vi "stage and voice coil synchronization.vi"() -> ()   [LabVIEW 2020]
uses:
  <vilib>/DAQmx/create/channels.llb/DAQmx Create Channel (CO-Pulse Generation-Frequency).vi
  <vilib>/DAQmx/configure/timing.llb/DAQmx Timing (Implicit).vi
  <vilib>/DAQmx/create/channels.llb/DAQmx Create Channel (AO-Voltage-Basic).vi
  <vilib>/measure/NI_MABase.lvlib
  <vilib>/DAQmx/write.llb/DAQmx Write (Analog 2D DBL NChan NSamp).vi
  <vilib>/DAQmx/configure/timing.llb/DAQmx Timing (Use Waveform).vi
panel:
  out "size(s) 2":i32
  out "size(s)":i32
  out "last value outside of loop":dbl
  out "number of samples written per channel":u32
  in  "stop":bool
  out "Waveform Graph":waveform(dbl)[](graph)
  out "Number of slices":dbl
  in  "End position (mm)":dbl
  out "last value inside of loop":dbl
  out "Total Z thickness (mm)":dbl
  in  "Z slice width (mm)":dbl
  in  "Start position(mm)":dbl
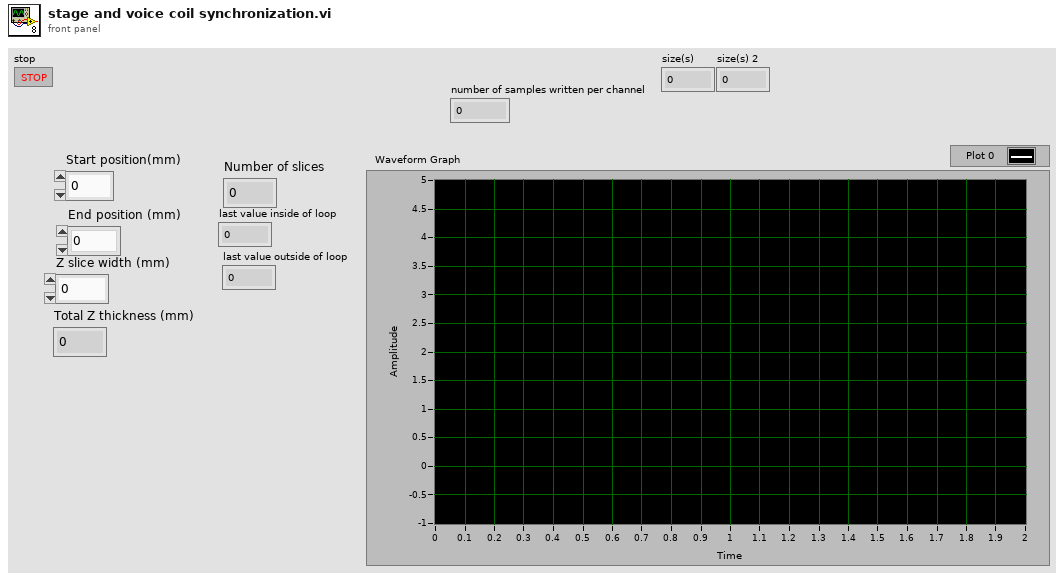
[diagram p1: front panel]
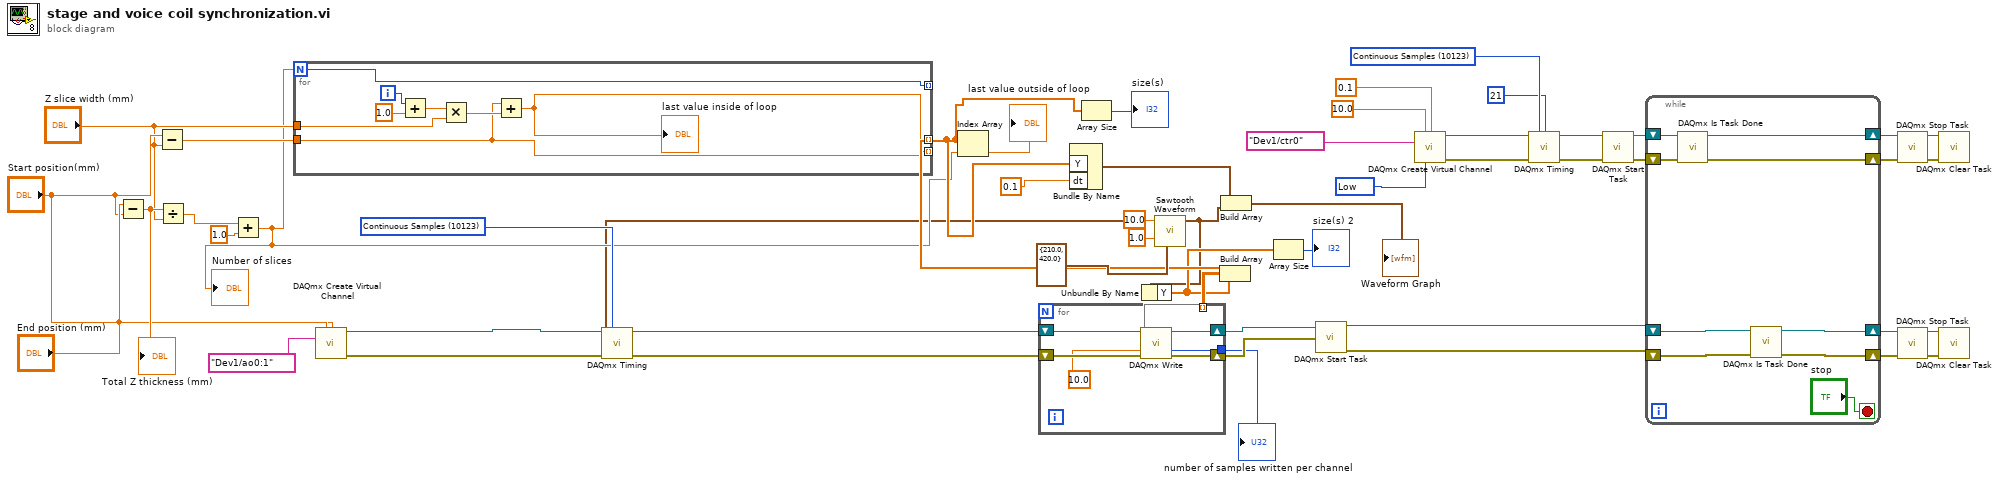
[diagram p0: block diagram]
diagram:
  w32 = 10214 items=["High"=10192, "Low"=10214] ("idle state")
  w34 = 10123 items=["Finite Samples"=10178, "Continuous Samples"=10123, "Hardware Timed Single Point"=12522] ("sample mode")
  w40 = 10123 items=["Finite Samples"=10178, "Continuous Samples"=10123, "Hardware Timed Single Point"=12522] ("sample mode")
  n1 = Subtract(x="End position (mm)", y="Start position(mm)") -> (x-y=w52:dbl)
  "Total Z thickness (mm)" <- w52
  n2 = Subtract(x="Start position(mm)", y="Z slice width (mm)") -> (x-y=w26:dbl)
  n3 = Divide(x=w52, y="Z slice width (mm)") -> (x/y=w5:dbl)
  n4 = Add(x=w5, y=1.0) -> (x+y=w2:dbl)
  "Number of slices" <- w2
  n5 = for {
    N: w2 -> [w55]
    tunnel: [w53] -> _ mode=indexing
    tunnel: "Z slice width (mm)" -> [w60]
    tunnel: [w54] -> w7 mode=indexing
    tunnel: [w55] -> _ mode=indexing
    tunnel: w26 -> [w53]
    i -> [w57]
    n6 = Add(x=w57, y=1.0) -> (x+y=w56:dbl)
    n7 = Multiply(x=w56, y=w60) -> (x*y=w59:dbl)
    n8 = Add(x=w53, y=w59) -> (x+y=w54:dbl)
    "last value inside of loop" <- w54
  }
  n9 = call-poly <vilib>:"DAQmx Create Virtual Channel.vi"("maximum value"="End position (mm)", "minimum value"="Start position(mm)", "physical channels"=tag "Dev1/ao0:1") -> ("task out"=w42:refnum<k21>, "error out"=w41:errorcluster)  [unwired: 11 in]
  n10 = Index Array "Index Array"(array=w7, index=w2) -> (element=→"last value outside of loop":dbl)
  n11 = Bundle By Name("Y"=w7, "dt"=0.1) -> (w14:waveform(dbl))  [unwired: 1 in]
  n12 = Array Size(array=w7) -> (size(s)=→"size(s)":i32)
  n13 = call <vilib>:"Sawtooth Waveform.vi"("sampling info"=cluster{"Fs":dbl, "#s":dbl} {"Fs"=210.0, "#s"=420.0}, "amplitude"=1.0, "frequency"=10.0) -> ("signal out"=w1:waveform(dbl))  [unwired: 7 in, 1 out]
  n14 = call-poly <vilib>:"DAQmx Timing.vi"("task/channels in"=w42, "sample mode"=w40, "waveform"=w1, "error in"=w41) -> ("task out"=w27:refnum<k21>, "error out"=w28:errorcluster)  [unwired: 10 in]
  n15 = Unbundle By Name(w1) -> ("Y"=w4:dbl[])
  n16 = Build Array(w7, w4) -> (w9:dbl[][])
  n17 = for {
    tunnel: [w62] -> w15
    tunnel: w9 -> [w61] mode=indexing
    shift-right: [w63] -> w16
    shift-left: w28 -> [w67]
    shift-right: [w64] -> w19
    shift-left: w27 -> [w66]
    n18 = call-poly <vilib>:"DAQmx Write.vi"("task/channels in"=w66, "data"=w61, "timeout"=10.0, "error in"=w67) -> ("task out"=w64:refnum<k21>, "number of samples written per channel"=w62:u32, "error out"=w63:errorcluster)  [unwired: 9 in]
  }
  "number of samples written per channel" <- w15
  n19 = Build Array(w14, w1) -> (→"Waveform Graph":waveform(dbl)[])
  n20 = Array Size(array=w4) -> (size(s)=→"size(s) 2":i32)
  n21 = call <vilib>:"DAQmx Start Task.vi"("task/channels in"=w19, "error in"=w16) -> ("task out"=w18:refnum<k21>, "error out"=w17:errorcluster)  [unwired: 12 in]
  n22 = call-poly <vilib>:"DAQmx Create Virtual Channel.vi"("frequency"=10.0, "duty cycle"=0.1, "counter"=tag "Dev1/ctr0", "idle state"=w32) -> ("task out"=w37:refnum<k21>, "error out"=w36:errorcluster)  [unwired: 10 in]
  n23 = call-poly <vilib>:"DAQmx Timing.vi"("task/channels in"=w37, "sample mode"=w34, "samples per channel"=21, "error in"=w36) -> ("task out"=w30:refnum<k21>, "error out"=w29:errorcluster)  [unwired: 10 in]
  n24 = call <vilib>:"DAQmx Start Task.vi"("task/channels in"=w30, "error in"=w29) -> ("task out"=w39:refnum<k21>, "error out"=w38:errorcluster)  [unwired: 12 in]
  n25 = while {
    shift-right: [w71] -> w44
    shift-left: w18 -> [w70]
    shift-right: [w74] -> w50
    shift-left: w39 -> [w76]
    shift-right: [w73] -> w48
    shift-left: w38 -> [w75]
    shift-right: [w72] -> w46
    shift-left: w17 -> [w69]
    stop <- "stop" stop-if-true
    n26 = call <vilib>:"DAQmx Is Task Done.vi"("task/channels in"=w76, "error in"=w75) -> ("task out"=w74:refnum<k21>, "error out"=w73:errorcluster)  [unwired: 11 in, 1 out]
    n27 = call <vilib>:"DAQmx Is Task Done.vi"("task/channels in"=w70, "error in"=w69) -> ("task out"=w71:refnum<k21>, "error out"=w72:errorcluster)  [unwired: 11 in, 1 out]
  }
  n28 = call <vilib>:"DAQmx Stop Task.vi"("task/channels in"=w50, "error in"=w48) -> ("task out"=w49:refnum<k21>, "error out"=w47:errorcluster)  [unwired: 12 in]
  n29 = call <vilib>:"DAQmx Stop Task.vi"("task/channels in"=w44, "error in"=w46) -> ("task out"=w43:refnum<k21>, "error out"=w45:errorcluster)  [unwired: 12 in]
  n30 = call <vilib>:"DAQmx Clear Task.vi"("task in"=w49, "error in"=w47) -> ()  [unwired: 13 in, 1 out]
  n31 = call <vilib>:"DAQmx Clear Task.vi"("task in"=w43, "error in"=w45) -> ()  [unwired: 13 in, 1 out]
